vi "MakeStetsonWindow.vi"(9 "radialsteps":i32, 10 "max radius":sgl, 11 "min radius":sgl) -> (3 "Halfstetson":dbl[](graph))   [LabVIEW 2011]
panel:
  in  "rise":sgl=5.0
  in  "fall":sgl=1.0
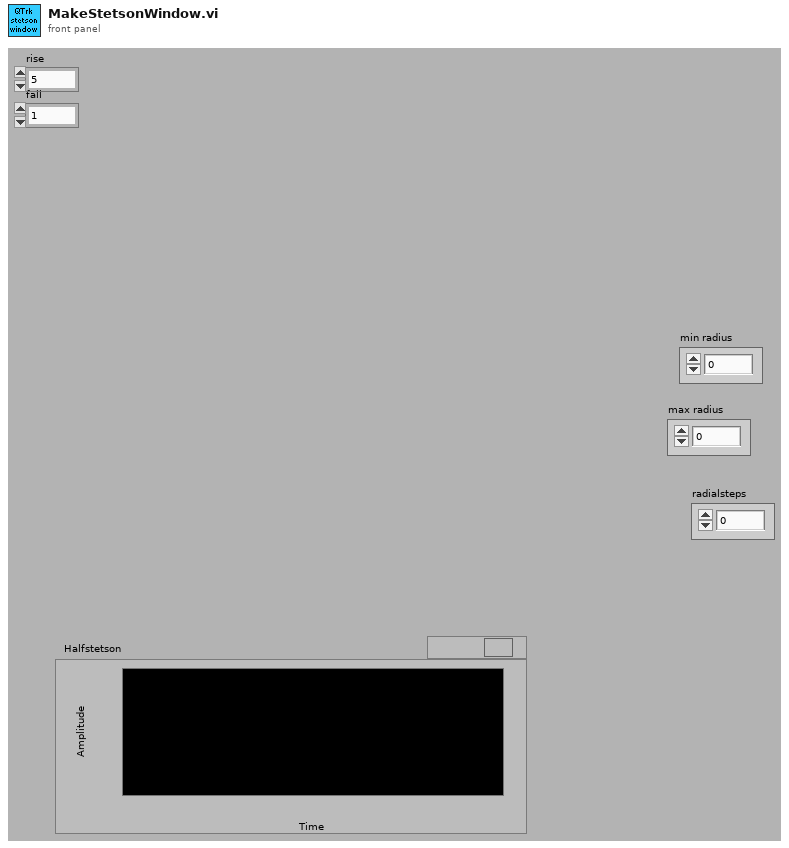
[diagram p1: front panel]
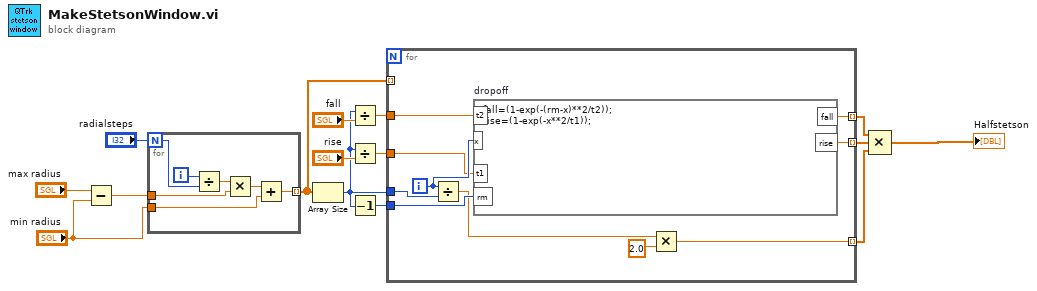
[diagram p0: block diagram]
diagram:
  n1 = Subtract(x="max radius", y="min radius") -> (x-y=w3:sgl)
  n2 = for {
    N: "radialsteps" -> [w21]
    tunnel: w3 -> [w19]
    tunnel: "min radius" -> [w17]
    tunnel: [w16] -> w1 mode=indexing
    i -> [w22]
    n3 = Divide(x=w22, y=w21) -> (x/y=w20:dbl)
    n4 = Multiply(x=w20, y=w19) -> (x*y=w18:dbl)
    n5 = Add(x=w18, y=w17) -> (x+y=w16:dbl)
  }
  n6 = Array Size(array=w1) -> (size(s)=w8:i32)
  n7 = Divide(x=w8, y="fall") -> (x/y=w12:sgl)
  n8 = Divide(x=w8, y="rise") -> (x/y=w13:sgl)
  n9 = Decrement(x=w8) -> (x-1=w7:i32)
  n10 = for {
    tunnel: w13 -> [w24]
    tunnel: w1 -> [_] mode=indexing
    tunnel: [w23] -> w10 mode=indexing
    tunnel: w12 -> [w30]
    tunnel: w7 -> [w32]
    tunnel: [w31] -> w11 mode=indexing
    tunnel: w8 -> [w28]
    tunnel: [w25] -> w9 mode=indexing
    i -> [w27]
    n11 = Divide(x=w27, y=w28) -> (x/y=w26:dbl)
    n12 = formula code="fall=(1-exp(-(rm-x)**2/t2));\nrise=(1-exp(-x**2/t1));" "dropoff"("x"=w27, "t2"=w30, "rm"=w32, "t1"=w24) -> ("fall"=w31:dbl, "rise"=w23:dbl)
    n13 = Multiply(x=w26, y=2.0) -> (x*y=w25:dbl)
  }
  n14 = Compound Arithmetic op=MULTIPLY(w11, w10, w9) -> (→"Halfstetson":dbl[])
